vi "conversion_inch_or_angle_to_microsteps.vi"(7 "Motor":u16(ring) items=["none", "1", "2", "3", "4", "all"], 10 "Inch/Angle":dbl) -> (2 "Microsteps":i32)   [LabVIEW 2013]
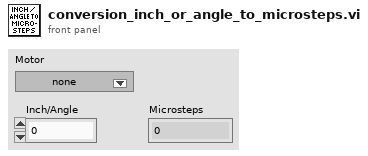
[diagram p1: front panel]
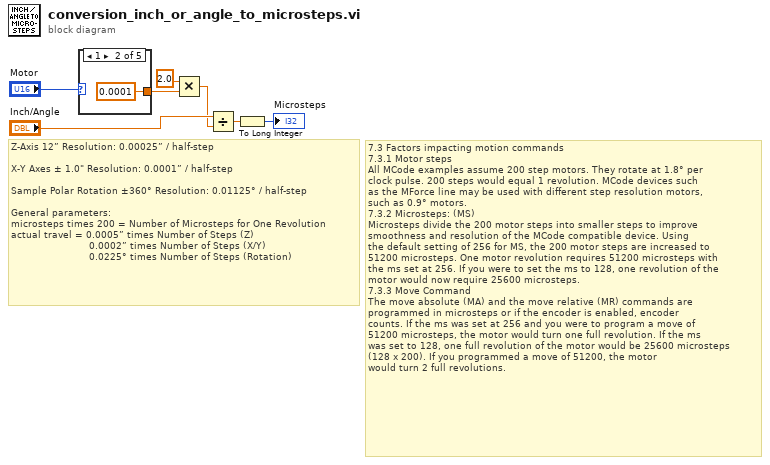
[diagram p0: block diagram]
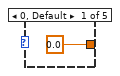
[diagram p2: hidden frame]
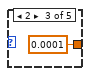
[diagram p3: hidden frame]
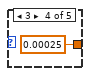
[diagram p4: hidden frame]
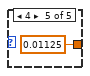
[diagram p5: hidden frame]
diagram:
  # "7.3 Factors impacting motion commands\n7.3.1 Motor steps\nAll MCode examples assume 200 step motors. They rotate at 1.8° per\nclock pulse. 200 steps would equal 1 revolution. MCode devices such\nas the MForce line may be used with different step resolution motors,\nsuch as 0.9° motors.\n7.3.2 Microsteps: (MS)\nMicrosteps divide the 200 motor steps into smaller steps to improve\nsmoothness and resolution of the MCode compatible device. Using\nthe default setting of 256 for MS, the 200 motor steps are increased to\n51200 microsteps. One motor revolution requires 51200 microsteps with\nthe ms set at 256. If you were to set the ms to 128, one revolution of the\nmotor would now require 25600 microsteps.\n7.3.3 Move Command\nThe move absolute (MA) and the move relative (MR) commands are\nprogrammed in microsteps or if the encoder is enabled, encoder\ncounts. If the ms was set at 256 and you were to program a move of\n51200 microsteps, the motor would turn one full revolution. If the ms\nwas set to 128, one full revolution of the motor would be 25600 microsteps\n(128 x 200). If you programmed a move of 51200, the motor\nwould turn 2 full revolutions."
  # "Z-Axis 12” Resolution: 0.00025” / half-step\n\nX-Y Axes ± 1.0\" Resolution: 0.0001” / half-step\n\nSample Polar Rotation ±360° Resolution: 0.01125° / half-step\n\nGeneral parameters:\nmicrosteps times 200 = Number of Microsteps for One Revolution\nactual travel = 0.0005” times Number of Steps (Z)\n                          0.0002” times Number of Steps (X/Y)\n                          0.0225° times Number of Steps (Rotation)"
  n1 = case shown="1" "Motor" {
    tunnel: [0.0 0.0001 0.0001 0.00025 0.01125] -> w6
    frame 0, Default {
    }
    frame 1 {
    }
    frame 2 {
    }
    frame 3 {
    }
    frame 4 {
    }
  }
  n2 = Multiply(x=2.0, y=w6) -> (x*y=w3:dbl)
  n3 = Divide(x="Inch/Angle", y=w3) -> (x/y=w2:dbl)
  n4 = To Long Integer(number=w2) -> (32bit integer=→"Microsteps":i32)
